vi "Write Label.vi"(8 "error in (no error)":errorcluster, 10 "Label":string, 11 "Column in":refnum<class "Column.lvclass">) -> (0 "error out":errorcluster, 3 "Column out":refnum<class "Column.lvclass">)   [LabVIEW 2013, in "Column.lvclass"]
uses:
  Column.lvclass
  Column.lvclass/Column.ctl
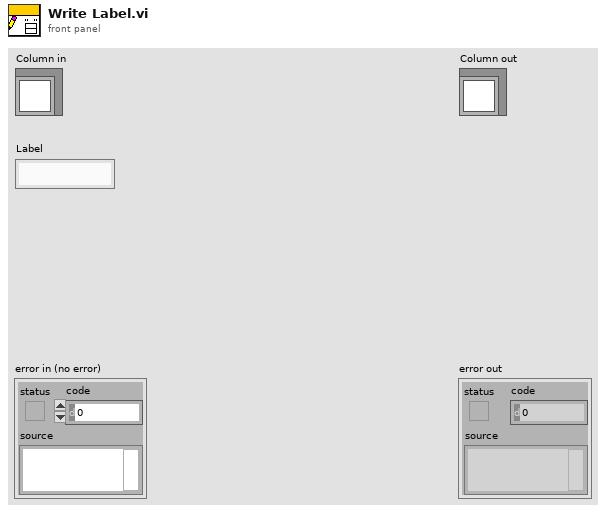
[diagram p1: front panel]
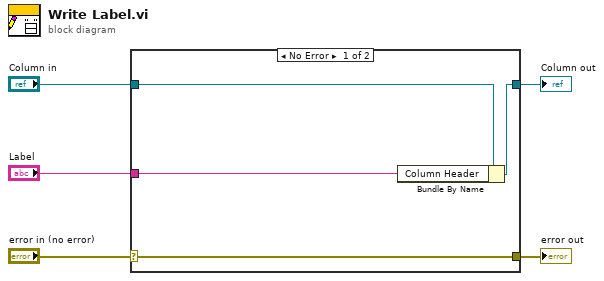
[diagram p0: block diagram]
diagram:
  n1 = case shown="No Error" "error in (no error)" {
    selector: "error in (no error)" -> [w9 w10]
    tunnel: [w9 w10] -> w4
    tunnel: [w7 w11] -> w2
    tunnel: "Column in" -> [w8 w11]
    tunnel: "Label" -> [w6 _]
    frame No Error {
      n2 = Bundle By Name(cluster=w8, "Column Header"=w6) -> (w7:refnum<class "Column.lvclass">)
    }
    frame Error {
    }
  }
  "error out" <- w4
  "Column out" <- w2
